vi "check tote alignment.vi"() -> ()   [LabVIEW 2014]
panel:
  out "distance from box":i32
  in  "distance":fxp<+/-,32,16>[](array[numeric])
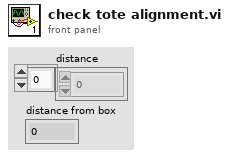
[diagram p1: front panel]
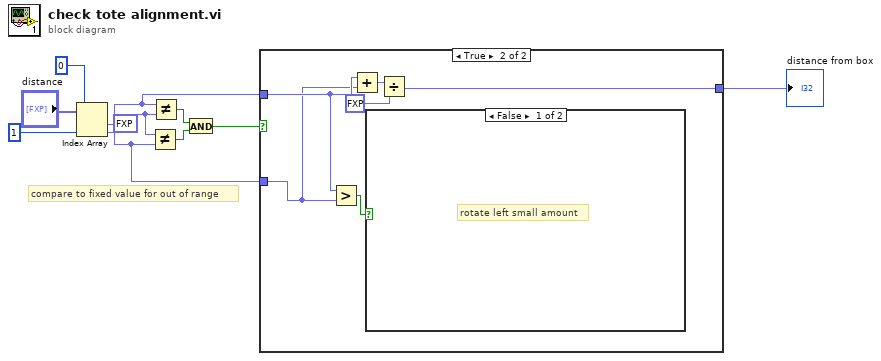
[diagram p0: block diagram]
diagram:
  w7 = fxp<+/-,32,16> 155.0 ("y")
  # "compare to fixed value for out of range"
  n1 = Index Array(array="distance", index #1=0 ("index"), index #2=1 ("index")) -> (element #1=w3:fxp<+/-,32,16>, element #2=w2:fxp<+/-,32,16>)
  n2 = Not Equal?(x=w7, y=w2) -> (x != y?=w6:bool)
  n3 = Not Equal?(x=w3, y=w7) -> (x != y?=w5:bool)
  n4 = And(x=w5, y=w6) -> (x .and. y?=w4:bool)
  n5 = case shown="True" w4 {
    tunnel: w3 -> [_ w15]
    tunnel: w2 -> [_ w14]
    tunnel: [_ w11] -> w1
    frame False {
    }
    frame True {
      n6 = Greater?(x=w15, y=w14) -> (0:w16:bool)
      n7 = Add(x=w15, y=w14) -> (x+y=w13:fxp<+/-,33,17>)
      n8 = case shown="False" w16 {
        frame False {
          # "rotate left small amount"
        }
        frame True {
          # "rotate right small amount"
        }
      }
      n9 = Divide(x=w13, y=fxp<+/-,33,17> 2.0) -> (x/y=w11:fxp<+/-,64,34>)
    }
  }
  "distance from box" <- w1
